vi "Begin.vi"() -> (0 "error out":errorcluster)   [LabVIEW 2013]
doc: "Called before other user functions, this VI is expected to open initial I/O refnums, load in file data, and do all program initialization. Notice that the <B>error out</B> terminal is simply used for data flow. Wiring it to other structures or subVIs ensures that this VI runs first."
uses:
  <vilib>/Rock Robotics/WPI/Joystick/WPI_JoystickDeviceEnum.ctl
  <vilib>/Rock Robotics/SystemInterfaces/Typedef/FPGA_TypedefDigitalModule.ctl
  <vilib>/Rock Robotics/SystemInterfaces/DIO/FPGA_DIOChannel.ctl
  <vilib>/Rock Robotics/SystemInterfaces/DIO/FPGA_DIORelayChannel.ctl
  <vilib>/Rock Robotics/SystemInterfaces/Typedef/FPGA_TypedefSolenoidModule.ctl
  <vilib>/Rock Robotics/WPI/Solenoid/WPI_SolenoidChannel.ctl
  <vilib>/Rock Robotics/SystemInterfaces/DIO/FPGA_DIOPWMChannel.ctl
  <vilib>/Rock Robotics/WPI/Encoder/WPI_EncoderType.ctl
  <vilib>/Rock Robotics/WPI/Solenoid/WPI_SolenoidValue.ctl
  <vilib>/Rock Robotics/WPI/Camera/WPI_CameraImageSize.ctl
  <vilib>/Rock Robotics/WPI/Camera/WPI_CameraWhite Balance Values.ctl
  <vilib>/Rock Robotics/WPI/Camera/WPI_CameraExposure Values.ctl
  <vilib>/Rock Robotics/WPI/Camera/WPI_CameraFrameRate.ctl
  <vilib>/Rock Robotics/WPI/Solenoid/WPI_SolenoidOpenDouble.vi
  <vilib>/Rock Robotics/WPI/Solenoid/WPI_SolenoidSetEnum.vi
  <vilib>/Rock Robotics/WPI/Counter/WPI_CounterDigitalInputToDigitalSource.vi
  <vilib>/Rock Robotics/WPI/RobotDrive/WPI_RobotDriveOpen2MotorWithVictor.vi
  <vilib>/Rock Robotics/WPI/MotorControl/WPI_MotorControlOpen Jaguar.vi
  <vilib>/Rock Robotics/WPI/MotorControl/WPI_MotorControlOpen Victor.vi
  <vilib>/Rock Robotics/WPI/Compressor/WPI_CompressorGetSetRefNum.vi
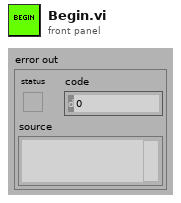
[diagram p1: front panel]
types:
  T1 = typedef "WPI_SolenoidValue.ctl" = enum16{"Off", "On", "Forward", "Reverse"}
  T2 = typedef "FPGA_DIOChannel.ctl" = enum8{"DIO 1", "DIO 2", "DIO 3", "DIO 4", "DIO 5", "DIO 6", "DIO 7", "DIO 8", "DIO 9", "DIO 10", "DIO 11", "DIO 12", "DIO 13", "DIO 14", "Invalid"}
  T3 = typedef "WPI_SolenoidChannel.ctl" = enum8{"Solenoid 1", "Solenoid 2", "Solenoid 3", "Solenoid 4", "Solenoid 5", "Solenoid 6", "Solenoid 7", "Solenoid 8", "Invalid"}
  T4 = typedef "FPGA_DIOPWMChannel.ctl" = enum8{"PWM 1", "PWM 2", "PWM 3", "PWM 4", "PWM 5", "PWM 6", "PWM 7", "PWM 8", "PWM 9", "PWM 10", "Invalid"}
  T5 = typedef "WPI_EncoderType.ctl" = enum16{"1x", "2x", "4x"}
  T6 = typedef "FPGA_TypedefSolenoidModule.ctl" = enum16{"Solenoid Module 1", "Solenoid Module 2"}
  T7 = typedef "FPGA_DIORelayChannel.ctl" = enum8{"Relay 1", "Relay 2", "Relay 3", "Relay 4", "Relay 5", "Relay 6", "Relay 7", "Relay 8", "Invalid"}
  T8 = typedef "WPI_JoystickDeviceEnum.ctl" = enum16{"USB 1", "USB 2", "USB 3", "USB 4", "Kinect 1", "Kinect 2"}
  T9 = typedef "FPGA_TypedefDigitalModule.ctl" = enum16{"Digital Module 1", "Digital Module 2"}
  T10 = typedef "WPI_CameraFrameRate.ctl" = u32
  T11 = typedef "WPI_CameraExposure Values.ctl" = enum16{"Auto", "Flicker-free 50 Hz", "Flicker-free 60 Hz", "Hold current"}
  T12 = typedef "WPI_CameraWhite Balance Values.ctl" = enum16{"Auto", "Fixed indoor", "Fixed outdoor 1", "Fixed outdoor 2", "Fixed fluorescent 1", "Fixed fluorescent 2", "Hold current"}
  T13 = typedef "WPI_CameraImageSize.ctl" = enum16{"640x480", "320x240", "160x120"}
  T14 = typedef "WPI_CameraDevRef.ctl" = cluster{"Camera Address":string, "CameraStatus":errorcluster, "Acquire Image Notifier":refnum<notifier>}
  T15 = typedef "WPI_DigitalInputDevRef.ctl" = cluster{"DevStatus":errorcluster, "DIO Channel":T2, "Digital Module":T9}
  T16 = typedef "WPI_MotorControlDeviceRef.ctl" = cluster{"DeviceStatus":errorcluster, "Type":enum16{"PWM", "CAN"}, "PWM":cluster{"Digital Module":T9, "PWM Channel":T4, "DeadBand":T17}, "CAN":cluster{"Device Number":u8, "Control Mode":T18, "Semaphore":T19, "Max Vout":dbl}, "Invert":bool, "TransformRef":T20, "InvTransformRef":T20}
  T17 = typedef "WPI_PWMDeadband.ctl" = cluster{"Name":string, "maxPositivePwm":i32, "minPositivePwm":i32, "centerPwm":i32, "maxNegativePwm":i32, "minNegativePwm":i32, "angularRange":u16}
  T18 = typedef "WPI_CANJaguar_ControlMode.ctl" = enum8{"Percent VBus", "Current", "Speed", "Position", "Voltage"}
  T19 = typedef "Semaphore RefNum" = refnum<k1>
  T20 = typedef "WPI_PWMTransform_ConPane.ctl" = refnum<vi>
  T21 = typedef "WPI_SolenoidDevRef.ctl" = cluster{"DevStatus":errorcluster, "Solenoid Module":T6, "Forward Solenoid Channel":T3, "Reverse Solenoid Channel":T3}
  T22 = typedef "FPGA_CounterEncoderSourceConvertionLVSourceType.ctl" = cluster{"DevStatus":errorcluster, "AnalogTriggerMode?":bool, "DigitalMode":cluster{"Digital Module":T9, "DIO Channel":T23}, "AnalogTriggerMode":cluster{"AnalogTriggerIndex":T24, "OutputType":T25}}
  T23 = typedef "FPGA_DIODigitalSourceChannel.ctl" = enum8{"DIO 1", "DIO 2", "DIO 3", "DIO 4", "DIO 5", "DIO 6", "DIO 7", "DIO 8", "DIO 9", "DIO 10", "DIO 11", "DIO 12", "DIO 13", "DIO 14", "Disabled"}
  T24 = typedef "FPGA_AnalogTriggerIndex.ctl" = enum8{"Trig 0", "Trig 1", "Trig 2", "Trig 3", "Trig 4", "Trig 5", "Trig 6", "Trig 7", "Invalid"}
  T25 = typedef "FPGA_AnalogTriggerOutType.ctl" = enum16{"InWindow", "TriggerState", "Rising", "Falling"}
  T26 = typedef "WPI_CompressorDevRef.ctl" = cluster{"DevStatus":errorcluster, "DigitalInputDevRef":T15, "RelayDevRef":T27}
  T27 = typedef "WPI_RelayDevRef.ctl" = cluster{"DevStatus":errorcluster, "Relay Channel":T7, "Digital Module":T9, "Relay Direction":T28}
  T28 = typedef "WPI_RelayDirection.ctl" = enum16{"Both directions", "Forward only", "Reverse only"}
  T29 = typedef "WPI_RobotDriveDevRef.ctl" = cluster{"DevStatus":errorcluster, "Motors[]":T16[], "Square Inputs":bool, "Max Output":dbl, "Isochronous":bool}
  T30 = typedef "WPI_EncoderDevRef.ctl" = cluster{"DevStatus":errorcluster, "EncoderIndex":T31, "CounterIndex":T32, "DistancePerCount":dbl, "Decoding Type":T5}
  T31 = typedef "FPGA_EncoderIdx.ctl" = enum8{"Enc 0", "Enc 1", "Enc 2", "Enc 3", "Invalid"}
  T32 = typedef "FPGA_CounterCtrSystemIndex.ctl" = enum8{"Ctr 0", "Ctr 1", "Ctr 2", "Ctr 3", "Ctr 4", "Ctr 5", "Ctr 6", "Ctr 7", "Invalid"}
  T33 = typedef "WPI_JoystickDevRef.ctl" = cluster{"Device":T8}
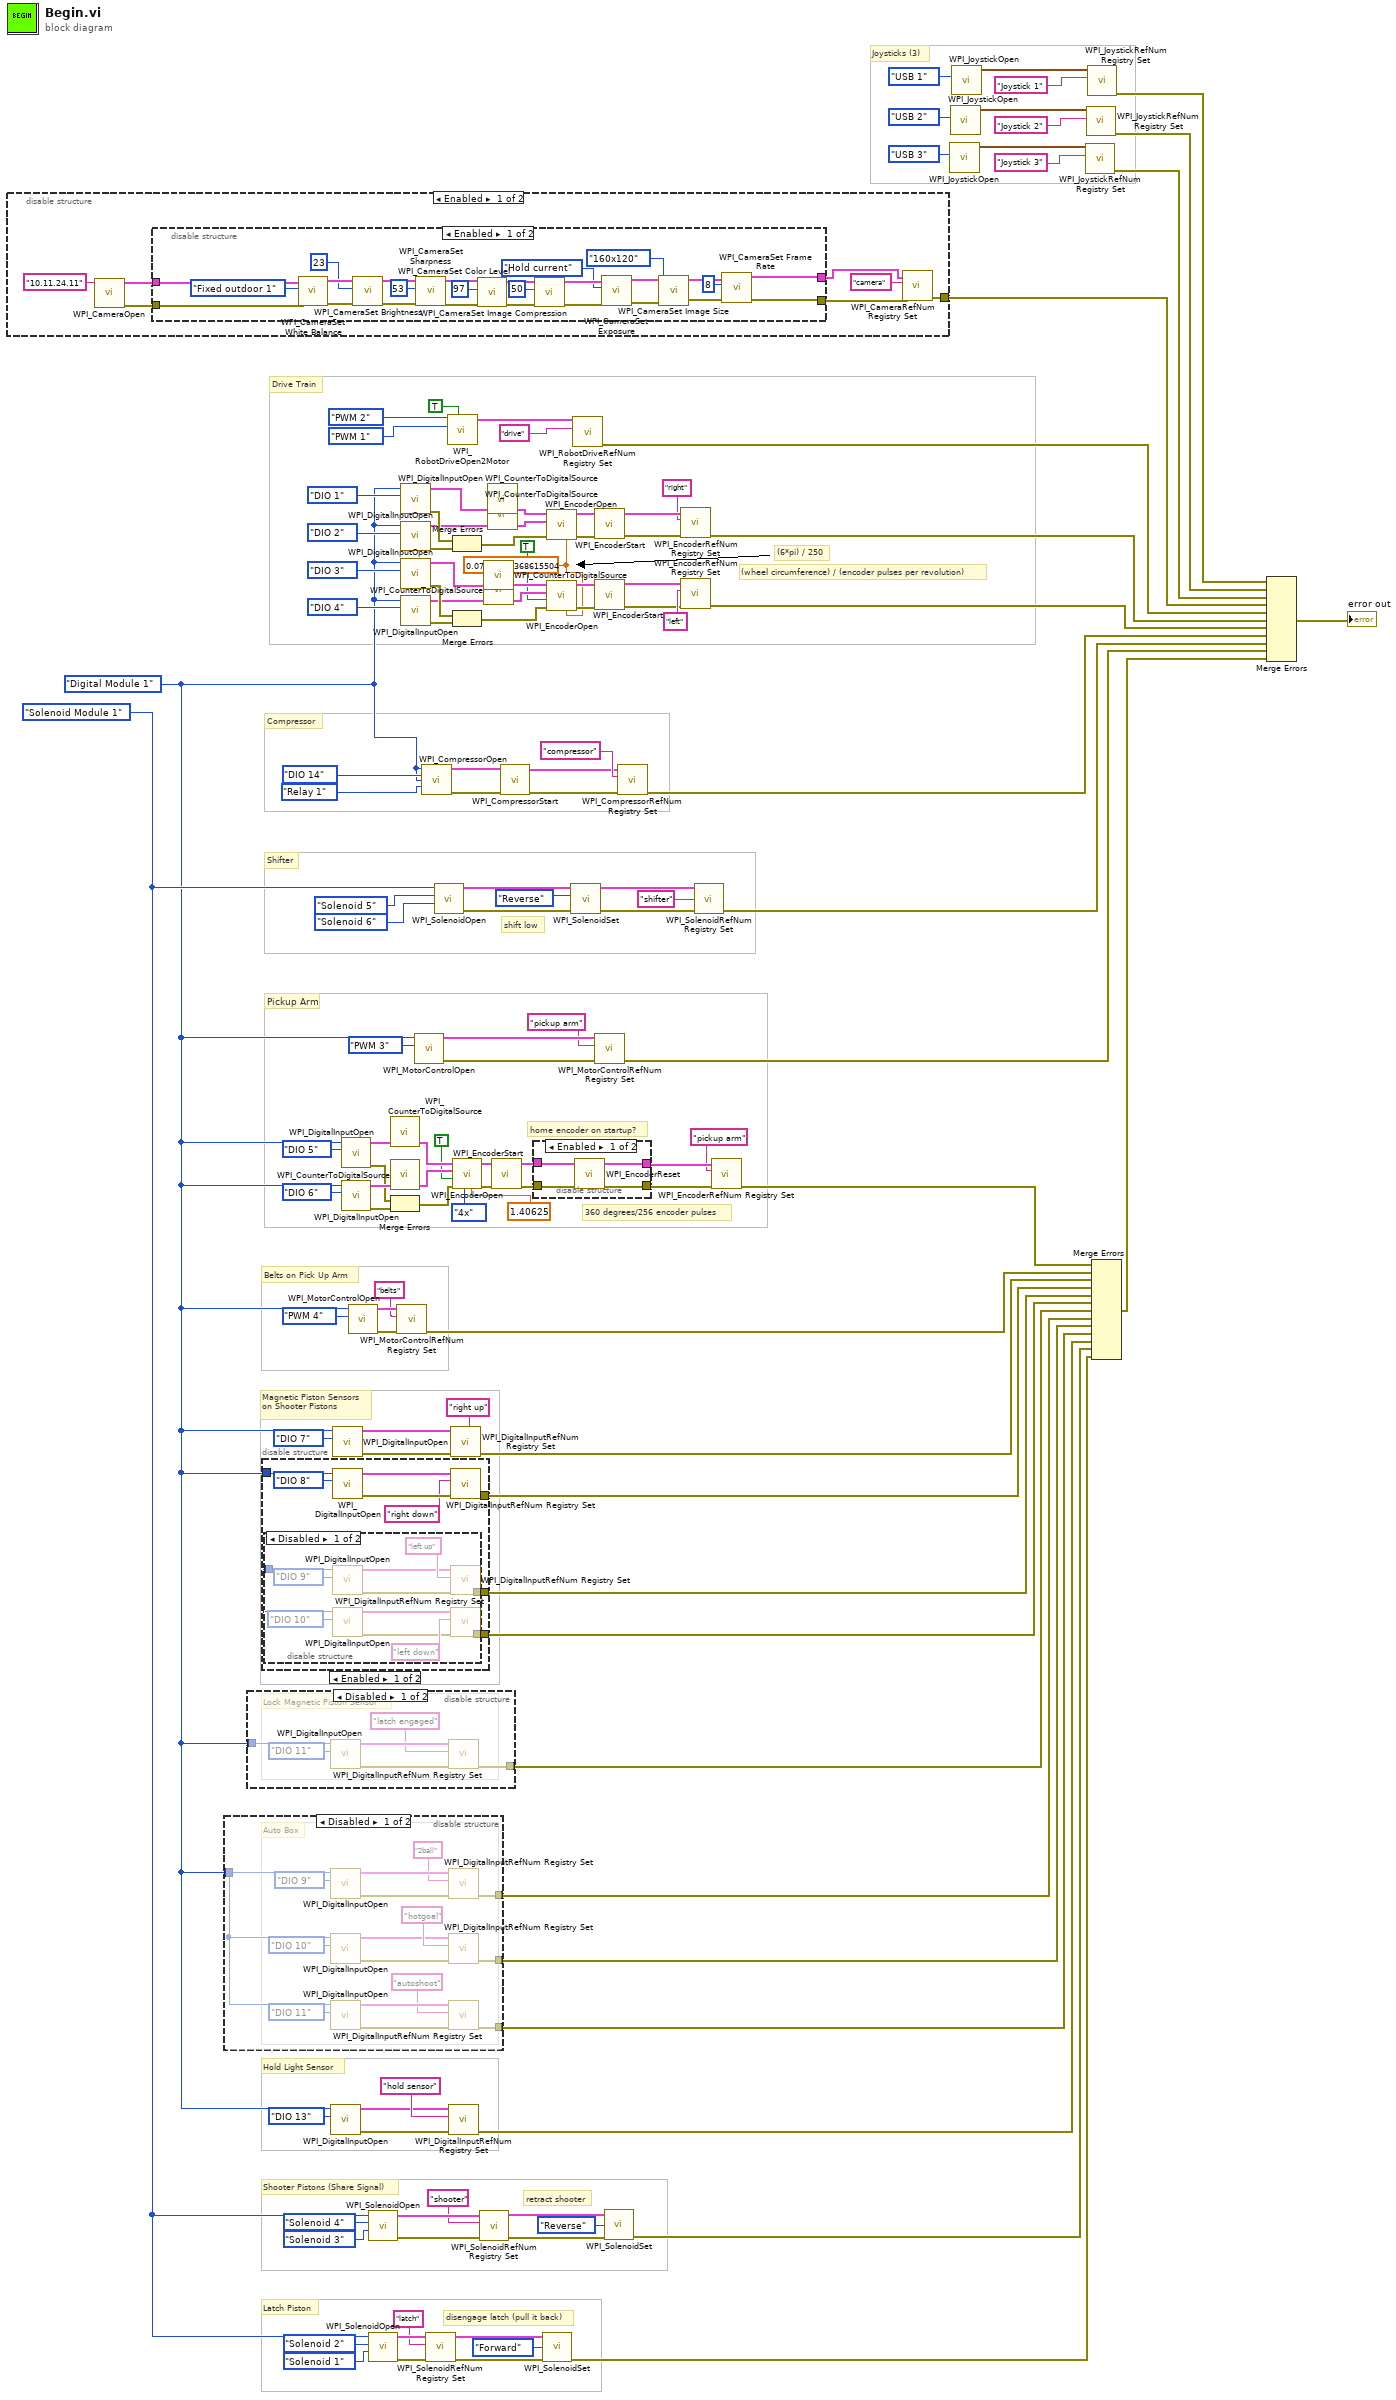
[diagram p0: block diagram]
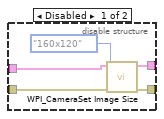
[diagram p4: hidden frame]
diagram:
  w81 = 0.07539822368615504 ("DistancePerCount")
  w24 = FPGA_TypedefSolenoidModule."Solenoid Module 1" ("Solenoid Module (Module 1)")
  w5 = FPGA_TypedefDigitalModule."Digital Module 1" ("Digital Module (Module 1)")
  # "retract shooter"
  # "disengage latch (pull it back)"
  # "360 degrees/256 encoder pulses"
  # "Hold Light Sensor"
  # "Joysticks (3)"
  # "Latch Piston"
  # "Shooter Pistons (Share Signal)"
  # "Magnetic Piston Sensors\non Shooter Pistons"
  # "Belts on Pick Up Arm"
  # "Pickup Arm"
  # "home encoder on startup?"
  # "Shifter"
  # "Compressor"
  # "Drive Train"
  # "shift low"
  # "(wheel circumference) / (encoder pulses per revolution)"
  # "(6*pi) / 250"
  n1 = disable-structure shown="Enabled" {
    disable-tunnel: [w144 _] -> w125
    frame Enabled {
      n2 = call <vilib>:"WPI_CameraOpen.vi"("Camera Address"="10.11.24.11") -> ("error out"=w139:errorcluster, "CameraDevRef"=w141:T14)  [unwired: 9 in]
      n3 = disable-structure shown="Enabled" {
        disable-tunnel: w141 -> [w168 w174]
        disable-tunnel: [w146 w173] -> w140
        disable-tunnel: w139 -> [w155 w172]
        disable-tunnel: [w145 w171] -> w138
        frame Enabled {
          n4 = call <vilib>:"WPI_CameraSet White Balance.vi"("error in (no error)"=w155, "White Balance"=WPI_CameraWhite_Balance_Values."Fixed outdoor 1", "CameraDevRef"=w168) -> ("error out"=w156:errorcluster, "CameraDevRef Out"=w167:T14)  [unwired: 7 in]
          n5 = call <vilib>:"WPI_CameraSet Brightness.vi"("error in (no error)"=w156, "Brightness"=23, "CameraDevRef"=w167) -> ("error out"=w157:errorcluster, "CameraDevRef Out"=w166:T14)  [unwired: 7 in]
          n6 = call <vilib>:"WPI_CameraSet Sharpness.vi"("error in (no error)"=w157, "Sharpness"=53, "CameraDevRef"=w166) -> ("error out"=w158:errorcluster, "CameraDevRef Out"=w165:T14)  [unwired: 7 in]
          n7 = call <vilib>:"WPI_CameraSet Color Level.vi"("error in (no error)"=w158, "Color Level"=97, "CameraDevRef"=w165) -> ("error out"=w159:errorcluster, "CameraDevRef Out"=w164:T14)  [unwired: 7 in]
          n8 = call <vilib>:"WPI_CameraSet Image Compression.vi"("error in (no error)"=w159, "Compression"=50, "CameraDevRef"=w164) -> ("error out"=w170:errorcluster, "CameraDevRef Out"=w169:T14)  [unwired: 7 in]
          n9 = call <vilib>:"WPI_CameraSet Exposure.vi"("error in (no error)"=w170, "Exposure"=WPI_CameraExposure_Values."Hold current", "CameraDevRef"=w169) -> ("error out"=w160:errorcluster, "CameraDevRef Out"=w163:T14)  [unwired: 7 in]
          n10 = call <vilib>:"WPI_CameraSet Image Size.vi"("error in (no error)"=w160, "Image Size"=WPI_CameraImageSize."160x120", "CameraDevRef"=w163) -> ("error out"=w161:errorcluster, "CameraDevRef Out"=w162:T14)  [unwired: 7 in]
          n11 = call <vilib>:"WPI_CameraSet Frame Rate.vi"("error in (no error)"=w161, "Frame Rate (fps)"=T10 8, "CameraDevRef"=w162) -> ("error out"=w145:errorcluster, "CameraDevRef Out"=w146:T14)  [unwired: 7 in]
        }
        frame Disabled {
          n12 = disable-structure shown="Enabled" {
            disable-tunnel: w172 -> [w178 w180]
            disable-tunnel: [w177 w180] -> w171
            disable-tunnel: w174 -> [w176 w181]
            disable-tunnel: [w175 w181] -> w173
            frame Disabled {
              n13 = call <vilib>:"WPI_CameraSet Image Size.vi"("error in (no error)"=w178, "Image Size"=WPI_CameraImageSize."160x120", "CameraDevRef"=w176) -> ("error out"=w177:errorcluster, "CameraDevRef Out"=w175:T14)  [unwired: 7 in]
            }
            frame Enabled {
            }
          }
        }
      }
      n14 = call <vilib>:"WPI_CameraRefNum Registry Set.vi"("error in (no error)"=w138, "refnum name"="camera", "CameraDevRef"=w140) -> ("error out"=w144:errorcluster)  [unwired: 7 in, 1 out]
    }
    frame Disabled {
    }
  }
  n15 = disable-structure shown="Disabled" {
    disable-tunnel: [w197 _] -> w13
    disable-tunnel: [w188 _] -> w6
    disable-tunnel: w5 -> [w183 _]
    disable-tunnel: [w182 _] -> w1
    frame Disabled {
      # "Auto Box"
      n16 = call <vilib>:"WPI_DigitalInputOpen.vi"("DIO Channel"=FPGA_DIOChannel."DIO 9", "Digital Module (Module 1)"=w183) -> ("error out"=w195:errorcluster, "DigitalInputDevRef"=w194:T15)  [unwired: 8 in]
      n17 = call <vilib>:"WPI_DigitalInputOpen.vi"("DIO Channel"=FPGA_DIOChannel."DIO 10", "Digital Module (Module 1)"=w183) -> ("error out"=w190:errorcluster, "DigitalInputDevRef"=w191:T15)  [unwired: 8 in]
      n18 = call <vilib>:"WPI_DigitalInputOpen.vi"("DIO Channel"=FPGA_DIOChannel."DIO 11", "Digital Module (Module 1)"=w183) -> ("error out"=w186:errorcluster, "DigitalInputDevRef"=w185:T15)  [unwired: 8 in]
      n19 = call <vilib>:"WPI_DigitalInputRefNum Registry Set.vi"("error in (no error)"=w195, "refnum name"="2ball", "DigitalInputDevRef"=w194) -> ("error out"=w197:errorcluster)  [unwired: 7 in, 1 out]
      n20 = call <vilib>:"WPI_DigitalInputRefNum Registry Set.vi"("error in (no error)"=w190, "refnum name"="hotgoal", "DigitalInputDevRef"=w191) -> ("error out"=w188:errorcluster)  [unwired: 7 in, 1 out]
      n21 = call <vilib>:"WPI_DigitalInputRefNum Registry Set.vi"("error in (no error)"=w186, "refnum name"="autoshoot", "DigitalInputDevRef"=w185) -> ("error out"=w182:errorcluster)  [unwired: 7 in, 1 out]
    }
    frame Enabled {
    }
  }
  n22 = disable-structure shown="Disabled" {
    disable-tunnel: w5 -> [w199 _]
    disable-tunnel: [w198 _] -> w17
    frame Disabled {
      # "Lock Magnetic Piston Sensor"
      n23 = call <vilib>:"WPI_DigitalInputOpen.vi"("DIO Channel"=FPGA_DIOChannel."DIO 11", "Digital Module (Module 1)"=w199) -> ("error out"=w202:errorcluster, "DigitalInputDevRef"=w201:T15)  [unwired: 8 in]
      n24 = call <vilib>:"WPI_DigitalInputRefNum Registry Set.vi"("error in (no error)"=w202, "refnum name"="latch engaged", "DigitalInputDevRef"=w201) -> ("error out"=w198:errorcluster)  [unwired: 7 in, 1 out]
    }
    frame Enabled {
      # "no latch magnetic sensor"
    }
  }
  n25 = disable-structure shown="Enabled" {
    disable-tunnel: [w208 _] -> w35
    disable-tunnel: w5 -> [w206 _]
    disable-tunnel: [w205 _] -> w19
    disable-tunnel: [w204 _] -> w18
    frame Enabled {
      n26 = disable-structure shown="Disabled" {
        disable-tunnel: w206 -> [w214 _]
        disable-tunnel: [w213 _] -> w205
        disable-tunnel: [w212 _] -> w204
        frame Disabled {
          n27 = call <vilib>:"WPI_DigitalInputOpen.vi"("DIO Channel"=FPGA_DIOChannel."DIO 9", "Digital Module (Module 1)"=w214) -> ("error out"=w215:errorcluster, "DigitalInputDevRef"=w216:T15)  [unwired: 8 in]
          n28 = call <vilib>:"WPI_DigitalInputOpen.vi"("DIO Channel"=FPGA_DIOChannel."DIO 10", "Digital Module (Module 1)"=w214) -> ("error out"=w217:errorcluster, "DigitalInputDevRef"=w218:T15)  [unwired: 8 in]
          n29 = call <vilib>:"WPI_DigitalInputRefNum Registry Set.vi"("error in (no error)"=w215, "refnum name"="left up", "DigitalInputDevRef"=w216) -> ("error out"=w213:errorcluster)  [unwired: 7 in, 1 out]
          n30 = call <vilib>:"WPI_DigitalInputRefNum Registry Set.vi"("error in (no error)"=w217, "refnum name"="left down", "DigitalInputDevRef"=w218) -> ("error out"=w212:errorcluster)  [unwired: 7 in, 1 out]
        }
        frame Enabled {
        }
      }
      n31 = call <vilib>:"WPI_DigitalInputOpen.vi"("DIO Channel"=FPGA_DIOChannel."DIO 8", "Digital Module (Module 1)"=w206) -> ("error out"=w211:errorcluster, "DigitalInputDevRef"=w210:T15)  [unwired: 8 in]
      n32 = call <vilib>:"WPI_DigitalInputRefNum Registry Set.vi"("error in (no error)"=w211, "refnum name"="right down", "DigitalInputDevRef"=w210) -> ("error out"=w208:errorcluster)  [unwired: 7 in, 1 out]
    }
    frame Disabled {
      # "dang, only one sensor\non the pistons..."
    }
  }
  n33 = call <vilib>:"WPI_DigitalInputOpen.vi"("DIO Channel"=FPGA_DIOChannel."DIO 13", "Digital Module (Module 1)"=w5) -> ("error out"=w21:errorcluster, "DigitalInputDevRef"=w22:T15)  [unwired: 8 in]
  n34 = call <vilib>:"WPI_DigitalInputOpen.vi"("DIO Channel"=FPGA_DIOChannel."DIO 7", "Digital Module (Module 1)"=w5) -> ("error out"=w40:errorcluster, "DigitalInputDevRef"=w39:T15)  [unwired: 8 in]
  n35 = call <vilib>:"WPI_DigitalInputOpen.vi"("DIO Channel"=FPGA_DIOChannel."DIO 5", "Digital Module (Module 1)"=w5) -> ("error out"=w57:errorcluster, "DigitalInputDevRef"=w62:T15)  [unwired: 8 in]
  n36 = call <vilib>:"WPI_DigitalInputOpen.vi"("DIO Channel"=FPGA_DIOChannel."DIO 6", "Digital Module (Module 1)"=w5) -> ("error out"=w58:errorcluster, "DigitalInputDevRef"=w61:T15)  [unwired: 8 in]
  n37 = call-poly <vilib>:"WPI_MotorControlOpen.vi"("PWM Channel"=FPGA_DIOPWMChannel."PWM 4", "Digital Module (Module 1)"=w5) -> ("error out"=w46:errorcluster, "MotorControlDeviceRef"=w45:T16)  [unwired: 8 in]
  n38 = call-poly <vilib>:"WPI_SolenoidOpen.vi"("Reverse Solenoid Channel"=WPI_SolenoidChannel."Solenoid 3", "Forward Solenoid Channel"=WPI_SolenoidChannel."Solenoid 4", "Solenoid Module (Module 1)"=w24) -> ("error out"=w30:errorcluster, "SolenoidDevRef"=w29:T21)  [unwired: 7 in]
  n39 = call-poly <vilib>:"WPI_SolenoidOpen.vi"("Reverse Solenoid Channel"=WPI_SolenoidChannel."Solenoid 1", "Forward Solenoid Channel"=WPI_SolenoidChannel."Solenoid 2", "Solenoid Module (Module 1)"=w24) -> ("error out"=w28:errorcluster, "SolenoidDevRef"=w27:T21)  [unwired: 7 in]
  n40 = call-poly <vilib>:"WPI_CounterToDigitalSource.vi"("DigitalInputDevRef"=w62) -> ("Digital Source"=w60:T22)  [unwired: 6 in]
  n41 = call-poly <vilib>:"WPI_CounterToDigitalSource.vi"("DigitalInputDevRef"=w61) -> ("Digital Source"=w59:T22)  [unwired: 6 in]
  n42 = Merge Errors(w57, w58) -> (w56:errorcluster)
  n43 = call <vilib>:"WPI_MotorControlRefNum Registry Set.vi"("error in (no error)"=w46, "refnum name"="belts", "MotorControlDevRef"=w45) -> ("error out"=w43:errorcluster)  [unwired: 7 in, 1 out]
  n44 = call <vilib>:"WPI_DigitalInputOpen.vi"("DIO Channel"=FPGA_DIOChannel."DIO 1", "Digital Module (Module 1)"=w5) -> ("error out"=w75:errorcluster, "DigitalInputDevRef"=w89:T15)  [unwired: 8 in]
  n45 = call <vilib>:"WPI_DigitalInputOpen.vi"("DIO Channel"=FPGA_DIOChannel."DIO 2", "Digital Module (Module 1)"=w5) -> ("error out"=w77:errorcluster, "DigitalInputDevRef"=w74:T15)  [unwired: 8 in]
  n46 = call <vilib>:"WPI_DigitalInputOpen.vi"("DIO Channel"=FPGA_DIOChannel."DIO 3", "Digital Module (Module 1)"=w5) -> ("error out"=w78:errorcluster, "DigitalInputDevRef"=w103:T15)  [unwired: 8 in]
  n47 = call <vilib>:"WPI_DigitalInputOpen.vi"("DIO Channel"=FPGA_DIOChannel."DIO 4", "Digital Module (Module 1)"=w5) -> ("error out"=w80:errorcluster, "DigitalInputDevRef"=w73:T15)  [unwired: 8 in]
  n48 = call-poly <vilib>:"WPI_MotorControlOpen.vi"("PWM Channel"=FPGA_DIOPWMChannel."PWM 3", "Digital Module (Module 1)"=w5) -> ("error out"=w69:errorcluster, "MotorControlDeviceRef"=w68:T16)  [unwired: 8 in]
  n49 = call <vilib>:"WPI_CompressorOpen.vi"("Pressure Switch Digital Module (Module 1)"=w5, "Pressure Switch DIO Channel"=FPGA_DIOChannel."DIO 14", "Relay Digital Module (Module 1)"=w5, "Relay Channel"=FPGA_DIORelayChannel."Relay 1") -> ("CompressorDevRef"=w117:T26, "error out"=w116:errorcluster)  [unwired: 10 in]
  n50 = call <vilib>:"WPI_SolenoidRefNum Registry Set.vi"("error in (no error)"=w28, "refnum name"="latch", "SolenoidDevRef"=w27) -> ("error out"=w15:errorcluster, "SolenoidDevRef"=w14:T21)  [unwired: 7 in]
  n51 = call-poly <vilib>:"WPI_SolenoidOpen.vi"("Reverse Solenoid Channel"=WPI_SolenoidChannel."Solenoid 6", "Forward Solenoid Channel"=WPI_SolenoidChannel."Solenoid 5", "Solenoid Module (Module 1)"=w24) -> ("error out"=w108:errorcluster, "SolenoidDevRef"=w109:T21)  [unwired: 7 in]
  n52 = call-poly <vilib>:"WPI_RobotDriveOpen2Motor.vi"("Left Motor Inverted"=TRUE, "Right Motor"=FPGA_DIOPWMChannel."PWM 1", "Left Motor"=FPGA_DIOPWMChannel."PWM 2") -> ("RobotDriveDevRef"=w105:T29)  [unwired: 7 in, 1 out]
  n53 = call <vilib>:"WPI_DigitalInputRefNum Registry Set.vi"("error in (no error)"=w21, "refnum name"="hold sensor", "DigitalInputDevRef"=w22) -> ("error out"=w2:errorcluster)  [unwired: 7 in, 1 out]
  n54 = call <vilib>:"WPI_DigitalInputRefNum Registry Set.vi"("error in (no error)"=w40, "refnum name"="right up", "DigitalInputDevRef"=w39) -> ("error out"=w36:errorcluster)  [unwired: 7 in, 1 out]
  n55 = Merge Errors(w75, w77) -> (w76:errorcluster)
  n56 = Merge Errors(w78, w80) -> (w79:errorcluster)
  n57 = call <vilib>:"WPI_EncoderOpen.vi"("DistancePerCount"=1.40625, "Decoding Type"=WPI_EncoderType."4x", "error in (no error)"=w56, "Invert Direction (False)"=TRUE, "BSource"=w59, "ASource"=w60) -> ("error out"=w55:errorcluster, "EncoderDevRef"=w54:T30)  [unwired: 4 in]
  n58 = call <vilib>:"WPI_SolenoidRefNum Registry Set.vi"("error in (no error)"=w30, "refnum name"="shooter", "SolenoidDevRef"=w29) -> ("error out"=w9:errorcluster, "SolenoidDevRef"=w10:T21)  [unwired: 7 in]
  n59 = call-poly <vilib>:"WPI_CounterToDigitalSource.vi"("DigitalInputDevRef"=w103) -> ("Digital Source"=w96:T22)  [unwired: 6 in]
  n60 = call-poly <vilib>:"WPI_CounterToDigitalSource.vi"("DigitalInputDevRef"=w73) -> ("Digital Source"=w97:T22)  [unwired: 6 in]
  n61 = call-poly <vilib>:"WPI_CounterToDigitalSource.vi"("DigitalInputDevRef"=w89) -> ("Digital Source"=w95:T22)  [unwired: 6 in]
  n62 = call-poly <vilib>:"WPI_CounterToDigitalSource.vi"("DigitalInputDevRef"=w74) -> ("Digital Source"=w94:T22)  [unwired: 6 in]
  n63 = call <vilib>:"WPI_EncoderStart.vi"("error in (no error)"=w55, "EncoderDevRef"=w54) -> ("error out"=w53:errorcluster, "EncoderDevRef"=w52:T30)  [unwired: 8 in]
  n64 = call <vilib>:"WPI_CompressorStart.vi"("error in (no error)"=w116, "CompressorDevRef"=w117) -> ("error out"=w115:errorcluster, "CompressorDevRef"=w114:T26)  [unwired: 8 in]
  n65 = disable-structure shown="Enabled" {
    disable-tunnel: w53 -> [w226 w227]
    disable-tunnel: w52 -> [w225 w228]
    disable-tunnel: [w224 w228] -> w50
    disable-tunnel: [w223 w227] -> w51
    frame Enabled {
      n66 = call <vilib>:"WPI_EncoderReset.vi"("error in (no error)"=w226, "EncoderDevRef"=w225) -> ("error out"=w223:errorcluster, "EncoderDevRef"=w224:T30)  [unwired: 8 in]
    }
    frame Disabled {
    }
  }
  n67 = call-poly <vilib>:"WPI_SolenoidSet.vi"("error in (no error)"=w15, "Value"=WPI_SolenoidValue."Forward", "SolenoidDevRef"=w14) -> ("error out"=w4:errorcluster)  [unwired: 7 in, 1 out]
  n68 = call <vilib>:"WPI_EncoderOpen.vi"("DistancePerCount"=w81, "error in (no error)"=w76, "BSource"=w94, "ASource"=w95) -> ("error out"=w93:errorcluster, "EncoderDevRef"=w92:T30)  [unwired: 6 in]
  n69 = call <vilib>:"WPI_EncoderOpen.vi"("DistancePerCount"=w81, "error in (no error)"=w79, "Invert Direction (False)"=TRUE, "BSource"=w97, "ASource"=w96) -> ("error out"=w98:errorcluster, "EncoderDevRef"=w99:T30)  [unwired: 5 in]
  n70 = call-poly <vilib>:"WPI_SolenoidSet.vi"("error in (no error)"=w108, "Value"=WPI_SolenoidValue."Reverse", "SolenoidDevRef"=w109) -> ("error out"=w107:errorcluster, "SolenoidDevRef"=w106:T21)  [unwired: 7 in]
  n71 = call <vilib>:"WPI_RobotDriveRefNum Registry Set.vi"("refnum name"="drive", "RobotDriveDevRef"=w105) -> ("error out"=w124:errorcluster)  [unwired: 8 in, 1 out]
  n72 = call <vilib>:"WPI_EncoderStart.vi"("error in (no error)"=w93, "EncoderDevRef"=w92) -> ("error out"=w91:errorcluster, "EncoderDevRef"=w90:T30)  [unwired: 8 in]
  n73 = call <vilib>:"WPI_EncoderStart.vi"("error in (no error)"=w98, "EncoderDevRef"=w99) -> ("error out"=w100:errorcluster, "EncoderDevRef"=w101:T30)  [unwired: 8 in]
  n74 = call <vilib>:"WPI_MotorControlRefNum Registry Set.vi"("error in (no error)"=w69, "refnum name"="pickup arm", "MotorControlDevRef"=w68) -> ("error out"=w65:errorcluster)  [unwired: 7 in, 1 out]
  n75 = call-poly <vilib>:"WPI_SolenoidSet.vi"("error in (no error)"=w9, "Value"=WPI_SolenoidValue."Reverse", "SolenoidDevRef"=w10) -> ("error out"=w3:errorcluster)  [unwired: 7 in, 1 out]
  n76 = call <vilib>:"WPI_CompressorRefNum Registry Set.vi"("error in (no error)"=w115, "refnum name"="compressor", "CompressorDevRef"=w114) -> ("error out"=w70:errorcluster)  [unwired: 7 in, 1 out]
  n77 = call <vilib>:"WPI_EncoderRefNum Registry Set.vi"("error in (no error)"=w91, "refnum name"="right", "EncoderDevRef"=w90) -> ("error out"=w123:errorcluster)  [unwired: 7 in, 1 out]
  n78 = call <vilib>:"WPI_EncoderRefNum Registry Set.vi"("error in (no error)"=w100, "refnum name"="left", "EncoderDevRef"=w101) -> ("error out"=w122:errorcluster)  [unwired: 7 in, 1 out]
  n79 = call <vilib>:"WPI_SolenoidRefNum Registry Set.vi"("error in (no error)"=w107, "refnum name"="shifter", "SolenoidDevRef"=w106) -> ("error out"=w71:errorcluster)  [unwired: 7 in, 1 out]
  n80 = call <vilib>:"WPI_EncoderRefNum Registry Set.vi"("error in (no error)"=w51, "refnum name"="pickup arm", "EncoderDevRef"=w50) -> ("error out"=w42:errorcluster)  [unwired: 7 in, 1 out]
  n81 = call <vilib>:"WPI_JoystickOpen.vi"("JoystickDevice"=WPI_JoystickDeviceEnum."USB 3") -> ("JoystickDevRef"=w136:T33)  [unwired: 10 in]
  n82 = call <vilib>:"WPI_JoystickOpen.vi"("JoystickDevice"=WPI_JoystickDeviceEnum."USB 2") -> ("JoystickDevRef"=w133:T33)  [unwired: 10 in]
  n83 = call <vilib>:"WPI_JoystickOpen.vi"("JoystickDevice"=WPI_JoystickDeviceEnum."USB 1") -> ("JoystickDevRef"=w130:T33)  [unwired: 10 in]
  n84 = call <vilib>:"WPI_JoystickRefNum Registry Set.vi"("refnum name"="Joystick 3", "JoystickDevRef"=w136) -> ("error out"=w126:errorcluster)  [unwired: 8 in, 1 out]
  n85 = call <vilib>:"WPI_JoystickRefNum Registry Set.vi"("refnum name"="Joystick 2", "JoystickDevRef"=w133) -> ("error out"=w127:errorcluster)  [unwired: 8 in, 1 out]
  n86 = call <vilib>:"WPI_JoystickRefNum Registry Set.vi"("refnum name"="Joystick 1", "JoystickDevRef"=w130) -> ("error out"=w128:errorcluster)  [unwired: 8 in, 1 out]
  n87 = Merge Errors(w42, w43, w36, w35, w19, w18, w17, w13, w6, w1, w2, w3, w4) -> (w41:errorcluster)
  n88 = Merge Errors(w128, w127, w126, w125, w124, w123, w122, w70, w71, w65, w41) -> (→"error out":errorcluster)
